vi "Calculatrice.vi"() -> ()   [LabVIEW 2024]
doc: "Calculatrice 2 -- ceci est un programme de calculatrice dans le cadre d'un exercise"
panel:
  out "Stockage Ope":T1(array[cluster])
  out "Array":T1(array[cluster])
  in  "error in (no error)":errorcluster
  in  "Test erreur":bool
  out "Gestion d'érreur":errorcluster
  in  "Btn_Stop":bool
  out "Screen":T2
  in  "Pad":T3
  # "Gestion des érreurs"
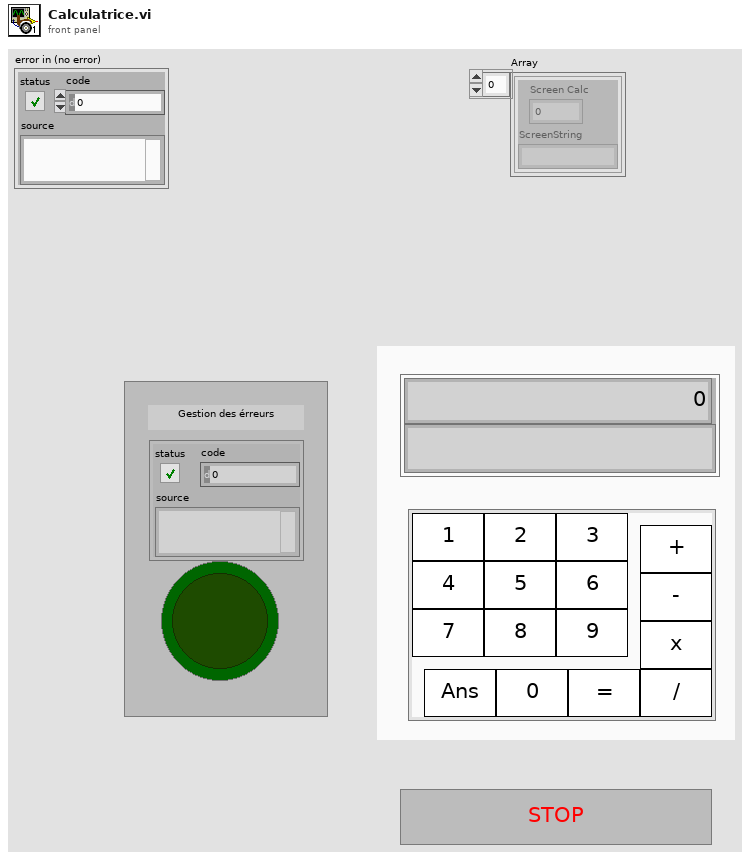
[diagram p1: front panel]
types:
  T1 = cluster{"Screen Calc":dbl, "ScreenString":string}[]
  T2 = cluster{"Screen Calc":dbl, "ScreenString":string}
  T3 = cluster{"1":bool, "2":bool, "Boolean 3":bool, "Boolean 4":bool, "Boolean 5":bool, "Boolean 6":bool, "Boolean 7":bool, "Boolean 8":bool, "Boolean 9":bool, "Boolean Zero":bool, "Moins":bool, "Multi":bool, "Plus":bool, "Div":bool, "Equal":bool, "Boolean Ans\nAns":bool}
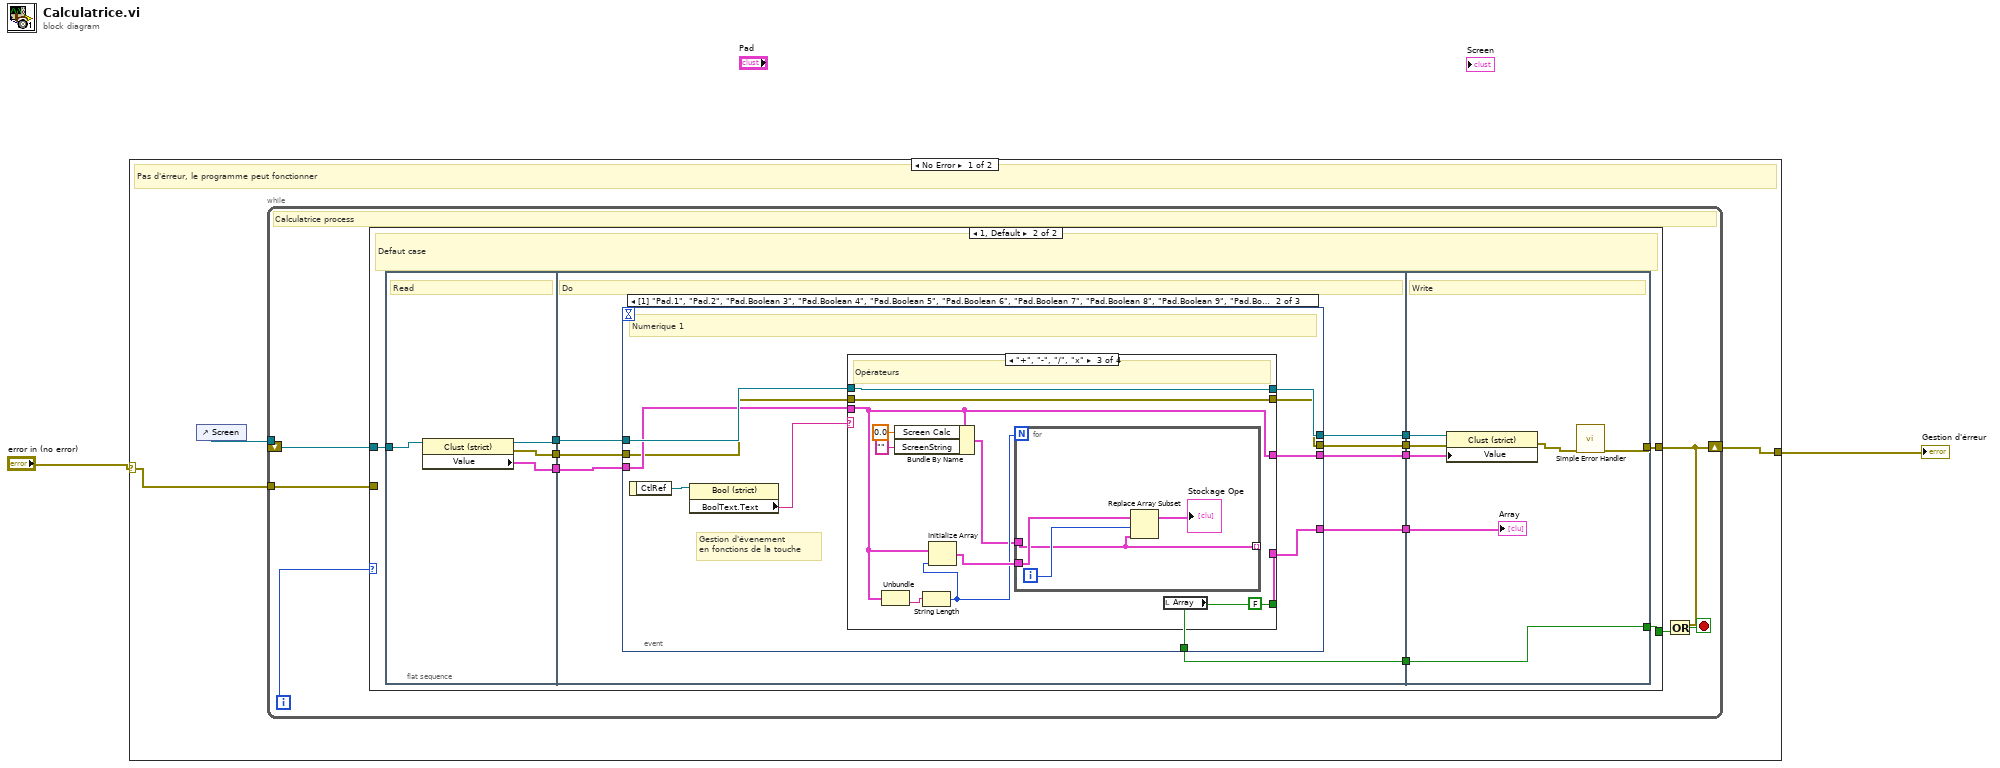
[diagram p0: block diagram]
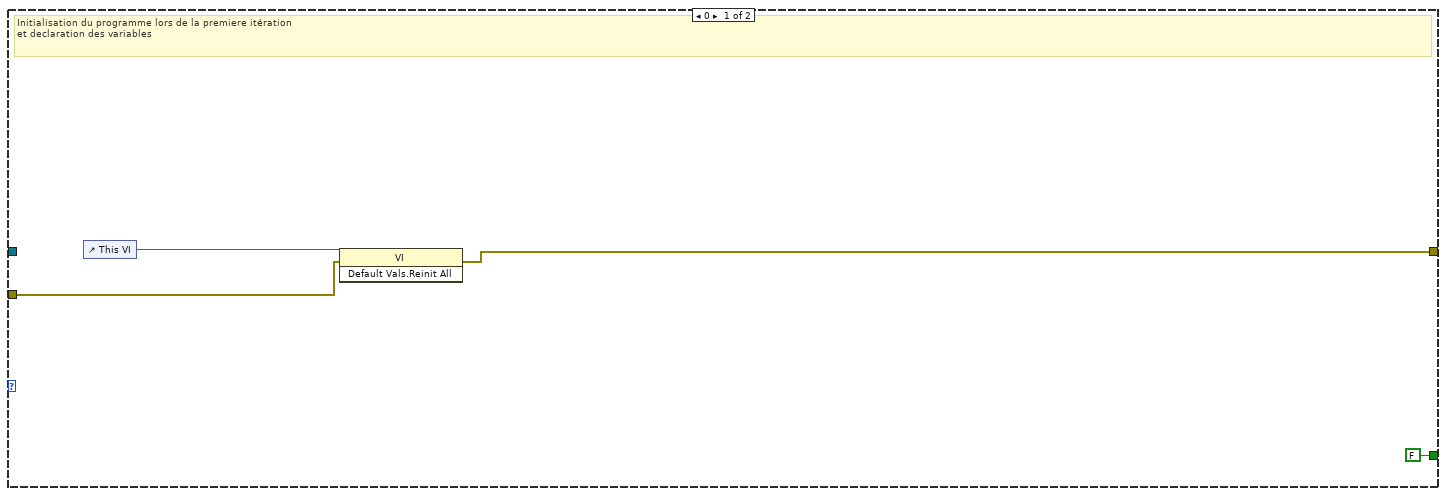
[diagram p2: hidden frame]
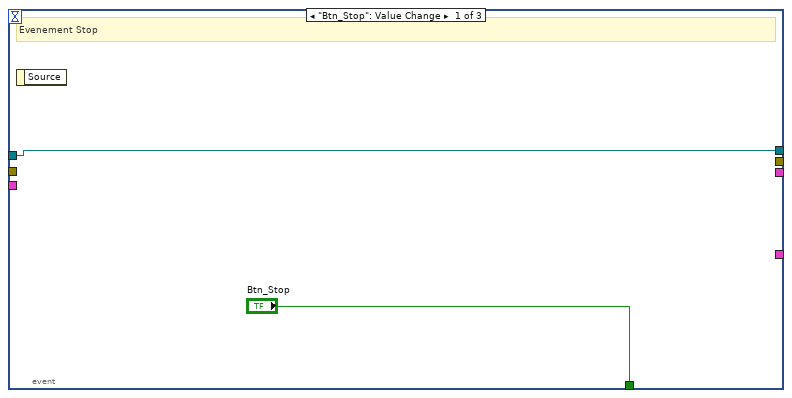
[diagram p3: hidden frame]
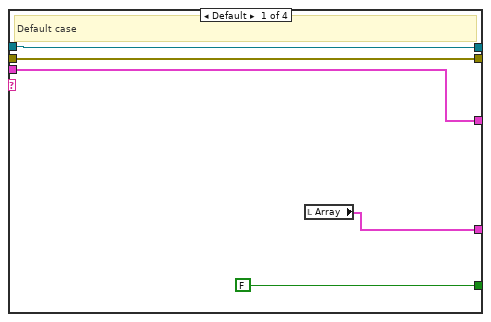
[diagram p4: hidden frame]
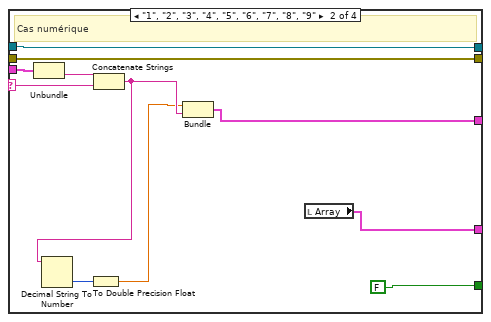
[diagram p5: hidden frame]
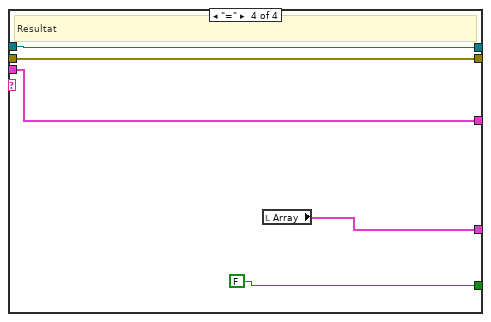
[diagram p6: hidden frame]
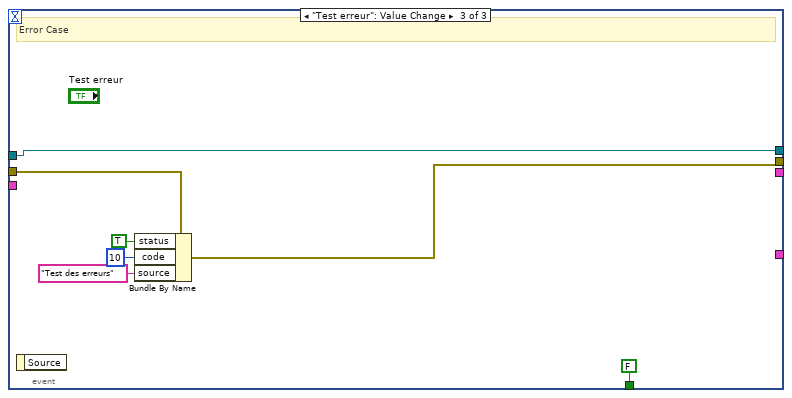
[diagram p7: hidden frame]
diagram:
  n1 = case shown="No Error" "error in (no error)" {
    selector: "error in (no error)" -> [w3 w101]
    tunnel: [w4 w101] -> w2
    frame No Error {
      # "Pas d'érreur, le programme peut fonctionner"
      n2 = control-ref of="Screen"() -> (w5:refnum<vi>)
      n3 = while {
        tunnel: w5 -> [w8]
        tunnel: w3 -> [w6]
        shift-right: [w9] -> w4
        shift-left: _ -> [_]
        i -> [w7]
        stop <- w10 stop-if-true
        # "Calculatrice process"
        n4 = case shown="1, Default" w7 {
          tunnel: [FALSE ("Btn_Stop") w20] -> w11
          tunnel: [w13 w19] -> w9
          tunnel: w8 -> [_ w18]
          tunnel: w6 -> [w15 _]
          frame 0 {
            # "Initialisation du programme lors de la premiere itération\net declaration des variables"
            n5 = control-ref of="This VI"() -> (w14:refnum<vi>)
            n6 = invoke class="VI" method="Default Vals.Reinit All"(reference=w14, error in=w15) -> (error out=w13:errorcluster)  [unwired: 1 in, 2 out]
          }
          frame 1, Default {
            # "Defaut case"
            n7 = flat-sequence {
              tunnel: [w29] -> w26
              tunnel: w18 -> [w30]
              tunnel: [w28] -> w25
              tunnel: [w27] -> w24
              tunnel: [w38] -> w23
              tunnel: w26 -> [w36]
              tunnel: [w35] -> w22
              tunnel: [w33] -> w21
              tunnel: w25 -> [w34]
              tunnel: w24 -> [w37]
              tunnel: [w32] -> w17
              tunnel: [w31] -> w16
              tunnel: [w100] -> w20
              tunnel: w23 -> [w100]
              tunnel: w22 -> [w99]
              tunnel: w21 -> [w98]
              tunnel: [w96] -> w19
              tunnel: w17 -> [w95]
              tunnel: w16 -> [w94]
              frame #0 {
                # "Read"
                n8 = property class="Clust (strict)"(reference=w30) -> (reference out=w29:refnum<vi>, error out=w28:errorcluster, "Value"=w27:T2)  [unwired: 1 in]
              }
              frame #1 {
                # "Do"
                n9 = event shown="[1] \"Pad.1\", \"Pad.2\", \"Pad.Boolean 3\", \"Pad.Boolean 4\", \"Pad.Boolean 5\", \"Pad.Boolean 6\", \"Pad.Boolean 7\", \"Pad.Boolean 8\", \"Pad.Boolean 9\", \"Pad.Boolean Zero\", \"Pad.Moins\", \"Pad.Multi\", \"Pad.Plus\", \"Pad.Div\", \"Pad.Equal\", \"Pad.Boolean Ans Ans\": Value Change" {
                  selector: _ -> [_ _ _]
                  dyn-events: _ -> [_ _ _]
                  timeout: _ -> [_ _ _]
                  tunnel: ["Btn_Stop" w48 FALSE ("Btn_Stop")] -> w38
                  tunnel: w37 -> [_ w45 _]
                  tunnel: w36 -> [w40 w47 w92]
                  tunnel: [w40 w46 w92] -> w35
                  tunnel: w34 -> [_ w44 w91]
                  tunnel: [_ w43 w87] -> w33
                  tunnel: [_ w42 _] -> w32
                  tunnel: [_ w41 _] -> w31
                  event "Btn_Stop": Value Change {
                    # "Evenement Stop"
                    n10 = event-data() -> ()  [unwired: 1 in, 1 out]
                  }
                  event "Pad.1", "Pad.2", "Pad.Boolean 3", "Pad.Boolean 4", "Pad.Boolean 5", "Pad.Boolean 6", "Pad.Boolean 7", "Pad.Boolean 8", "Pad.Boolean 9", "Pad.Boolean Zero", "Pad.Moins", "Pad.Multi", "Pad.Plus", "Pad.Div", "Pad.Equal", "Pad.Boolean Ans\nAns": Value Change {
                    # "Gestion d'évenement\nen fonctions de la touche"
                    # "Numerique 1"
                    n11 = event-data() -> ("CtlRef"=w50:refnum<vi>)  [unwired: 1 in]
                    n12 = property on="Property Node" class="Bool (strict)"(reference=w50) -> ("BoolText.Text"=w49:string)  [unwired: 1 in, 2 out]
                    n13 = case shown="\"+\", \"-\", \"/\", \"x\"" w49 {
                      selector: w49 -> [_ w62 _ _]
                      tunnel: [FALSE FALSE FALSE FALSE] -> w48
                      tunnel: w45 -> [w51 w61 w67 w82]
                      tunnel: w47 -> [w54 w65 w76 w85]
                      tunnel: [w54 w65 w76 w85] -> w46
                      tunnel: w44 -> [w53 w63 w75 w84]
                      tunnel: [w53 w63 w75 w84] -> w43
                      tunnel: [w52 w57 w68 w83] -> w42
                      tunnel: [w51 w56 w67 w82] -> w41
                      frame Default {
                        # "Default case"
                        n14 = local read "Array"() -> (w52:T1)
                      }
                      frame "1", "2", "3", "4", "5", "6", "7", "8", "9" {
                        # "Cas numérique"
                        n15 = Unbundle(w61) -> ("ScreenString"=w60:string)  [unwired: 1 out]
                        n16 = Concatenate Strings(w60, w62) -> (w59:string)
                        n17 = Decimal String To Number(string=w59) -> (number=w64:i32)  [unwired: 2 in, 1 out]
                        n18 = To Double Precision Float(number=w64) -> (double precision float=w58:dbl)
                        n19 = Bundle(w58, w59) -> (w56:cluster{dbl, string})  [unwired: 1 in]
                        n20 = local read "Array"() -> (w57:T1)
                      }
                      frame "+", "-", "/", "x" {
                        # "Opérateurs"
                        n21 = Unbundle(w67) -> ("ScreenString"=w74:string)  [unwired: 1 out]
                        n22 = Bundle By Name(cluster=w67, "Screen Calc"=0.0, "ScreenString"="") -> (w69:T2)
                        n23 = String Length(string=w74) -> (length=w70:i32)
                        n24 = Initialize Array "Initialize Array"(w67, w70) -> (w71:T1)
                        n25 = for {
                          N: w70 -> [_]
                          tunnel: w71 -> [w81]
                          tunnel: [w78] -> _ mode=indexing
                          tunnel: w69 -> [w78]
                          i -> [w80]
                          n26 = Replace Array Subset(array=w81, new element=w78, index=w80) -> (→"Stockage Ope":T1)
                        }
                        n27 = local read "Array"() -> (w68:T1)
                      }
                      frame "=" {
                        # "Resultat"
                        n28 = local read "Array"() -> (w83:T1)
                      }
                    }
                  }
                  event "Test erreur": Value Change {
                    # "Error Case"
                    n29 = event-data() -> ()  [unwired: 1 in, 1 out]
                    n30 = Bundle By Name(cluster=w91, "status"=TRUE, "code"=10, "source"="Test des erreurs") -> (w87:errorcluster)
                  }
                }
              }
              frame #2 {
                # "Write"
                n31 = property class="Clust (strict)"(reference=w99, error in=w98, "Value"=w94) -> (error out=w97:errorcluster)  [unwired: 1 out]
                n32 = call <vilib>:"Simple Error Handler.vi"("error in (no error)"=w97) -> ("error out"=w96:errorcluster)  [unwired: 4 in, 4 out]
                "Array" <- w95
              }
            }
          }
        }
        n33 = Or(x=w9, y=w11) -> (x .or. y?=w10:bool)
      }
    }
    frame Error {
    }
  }
  "Gestion d'érreur" <- w2
